vi "SLL DE Get DO Safe Values form INI File.vi"(8 "error in (no error)":errorcluster) -> (0 "error out":errorcluster, 1 "DO Safe Values":bool[](array[boolean]), 2 "DO Channel Names (String)":string[](array[string]), 3 "DO Channels (Enum)":T1[](array[typedef]))   [LabVIEW 2013]
doc: "Copyright © 2005, Soliton Technologies.\nAll rights reserved."
uses:
  Controls/SLL DE List of Digital Outputs.ctl
  Controls/SLL DE DAQ Parameters LV2Global Options.ctl
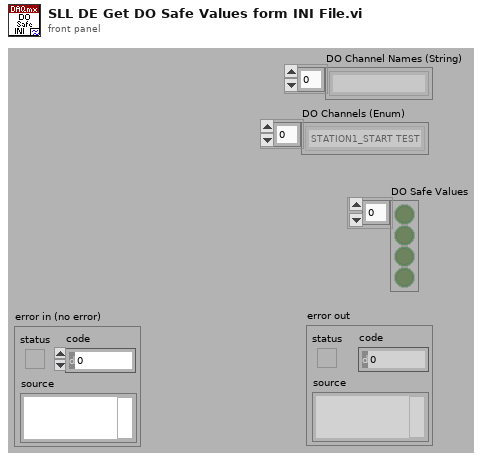
[diagram p1: front panel]
types:
  T1 = typedef "SLL DE List of Digital Outputs.ctl" = enum16{"STATION1_START TEST", "STATION1_STOP TEST", "STATION1_LIGHT1", "STATION1_LIGHT2", "STATION1_LIGHT3", "STATION1_SELECT_TEST", "STATION2_START TEST", "STATION2_STOP TEST", "STATION2_LIGHT1", "STATION2_LIGHT2", "STATION2_LIGHT3", "STATION2_SELECT_TEST", "STATION3_START TEST", "STATION3_STOP TEST", "STATION3_LIGHT1", "STATION3_LIGHT2", "STATION3_LIGHT3", "STATION3_SELECT_TEST", "STATION4_START TEST", "STATION4_STOP TEST", "STATION4_LIGHT1", "STATION4_LIGHT2", "STATION4_LIGHT3", "STATION4_SELECT_TEST"}
  T2 = typedef "SLL DE DAQ Parameters LV2Global Options.ctl" = enum16{"Read", "Write"}
  T3 = typedef "SLL DE DAQ Engine Parameters.ctl" = cluster{"Enable Engines":cluster{"AI Enable":bool, "AO Enable":bool, "DI Enable":bool, "DO Enable":bool}, "DAQ Control Type":cluster{"Analog Input":enum16{"Finite", "Continuous", "Driver"}, "Analog Output":enum16{"Finite", "Continuous", "Driver"}, "Digital Input":enum16{"Finite", "Continuous", "Driver"}, "Digital Output":enum16{"Finite", "Continuous", "Driver"}}, "DAQ Parameters":cluster{"AI Sampling Rate (Samples/Sec)":dbl, "MvgAVG Window Size (# of Points)":i32, "Enable Filter":bool, "Enable MvgAVG":bool, "Circular Buffer Size (Sec)":dbl, "AO Sampling Rate (Samples/Sec)":dbl, "Graph Update Rate (Samples/Sec)":dbl, "File Logging Rate (Samples/Sec)":i32}, "AO Safe Values":cluster{"Analog Outputs Name":T4, "Analog Outputs Safe Value":dbl}[], "DO Safe Values":cluster{"Digital Outputs Name":T1, "Digital Outputs Safe Value":bool}[], "DO Interconnected Lines":cluster{"First DO Line":string, "Second DO Line":string}[], "AI Channels Unit":cluster{"Channel Name":T5, "Channel Type":T6}[], "Units Information":cluster{"Channel Type":T6, "Unit Text":string, "Maximum":dbl, "Minmum":dbl, "Increments":dbl}[]}
  T4 = typedef "SLL DE List of Analog Outputs.ctl" = enum16{"None"}
  T5 = typedef "SLL DE List of Analog Inputs.ctl" = enum16{"None"}
  T6 = typedef "SLL DE List of AI Channel Type.ctl" = enum16{"Pressure", "Flow", "Temperature", "Time Scale", "Voltage", "Current", "Frequency", "Sound", "Speed", "Torque", "Distance", "Channel Type 1", "Channel Type 2", "Channel Type 3"}
  T7 = cluster{"Digital Outputs Name":T1, "Digital Outputs Safe Value":bool}[]
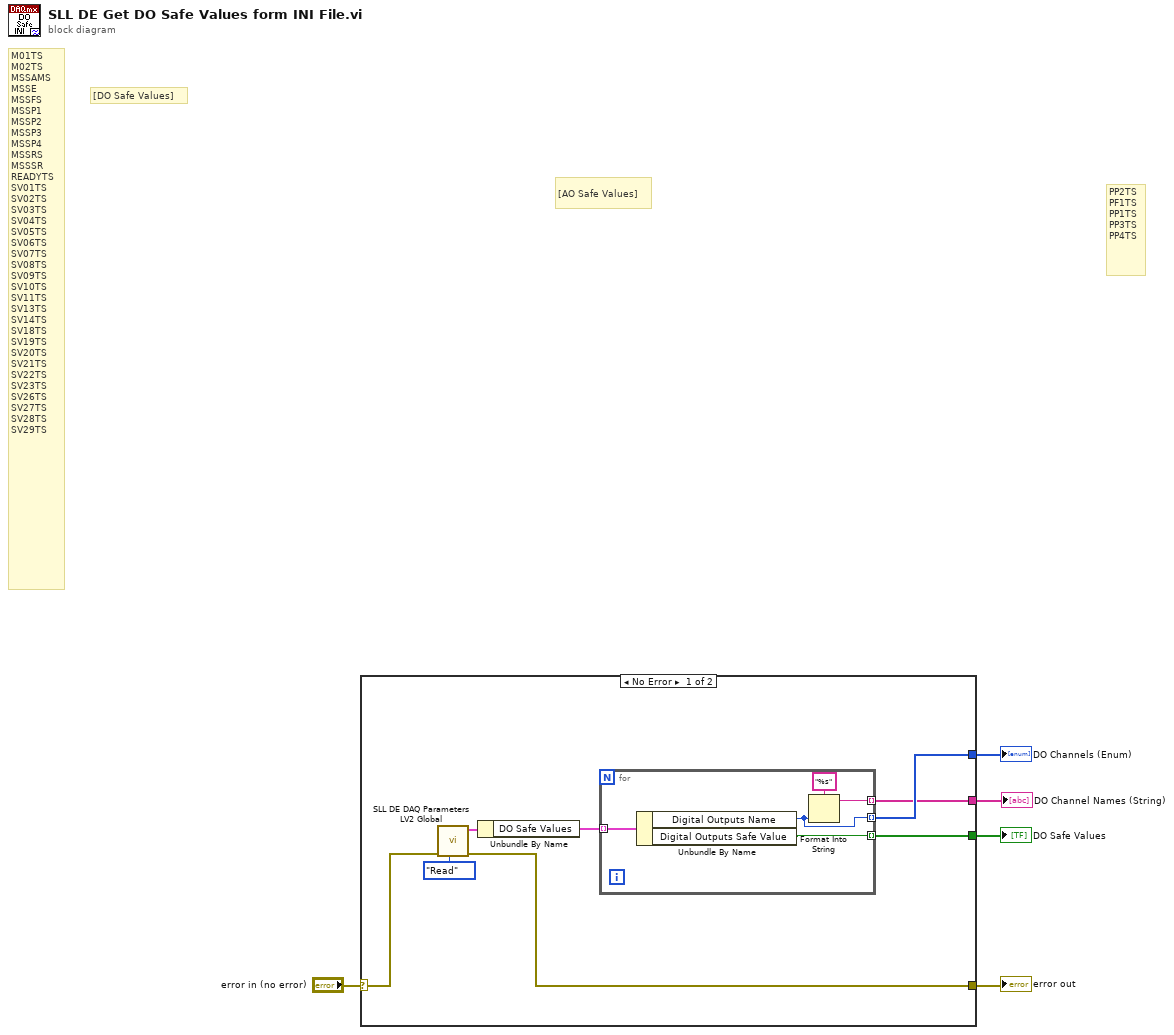
[diagram p0: block diagram]
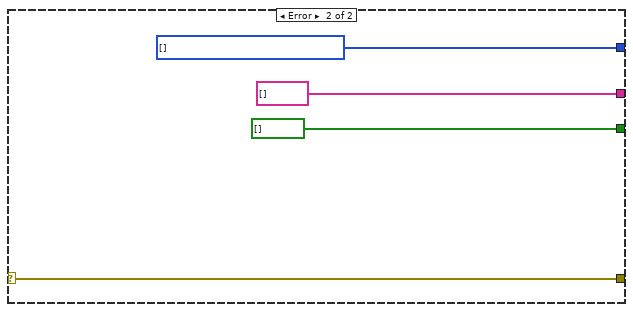
[diagram p2: hidden frame]
diagram:
  # "[DO Safe Values]"
  # "PP2TS\nPF1TS\nPP1TS\nPP3TS\nPP4TS"
  # "[AO Safe Values]"
  # "M01TS\nM02TS\nMSSAMS\nMSSE\nMSSFS\nMSSP1\nMSSP2\nMSSP3\nMSSP4\nMSSRS\nMSSSR\nREADYTS\nSV01TS\nSV02TS\nSV03TS\nSV04TS\nSV05TS\nSV06TS\nSV07TS\nSV08TS\nSV09TS\nSV10TS\nSV11TS\nSV13TS\nSV14TS\nSV18TS\nSV19TS\nSV20TS\nSV21TS\nSV22TS\nSV23TS\nSV26TS\nSV27TS\nSV28TS\nSV29TS"
  n1 = case shown="No Error" "error in (no error)" {
    selector: "error in (no error)" -> [w13 w22]
    tunnel: [w12 w22] -> w4
    tunnel: [w11 bool[] [] ("Key Values")] -> w3
    tunnel: [w10 w20] -> w2
    tunnel: [w9 string[] []] -> w1
    frame No Error {
      n2 = call "SLL DE DAQ Parameters LV2 Global.vi"("Option"=SLL_DE_DAQ_Parameters_LV2Global_Options."Read", "Error in (no error)"=w13) -> ("Error out"=w12:errorcluster, "Global Info"=w7:T3)  [unwired: 8 in]
      n3 = Unbundle By Name(w7) -> ("DO Safe Values"=w8:T7)
      n4 = for {
        tunnel: w8 -> [w18] mode=indexing
        tunnel: [w16] -> w11 mode=indexing
        tunnel: [w15] -> w10 mode=indexing
        tunnel: [w14] -> w9 mode=indexing
        n5 = Unbundle By Name(w18) -> ("Digital Outputs Name"=w15:T1, "Digital Outputs Safe Value"=w16:bool)
        n6 = Format Into String(format string="%s", w15) -> (resulting string=w14:string)  [unwired: 2 in, 1 out]
      }
    }
    frame Error {
      w20 = T1[] [] items=["STATION1_START TEST", "STATION1_STOP TEST", "STATION1_LIGHT1", "STATION1_LIGHT2", "STATION1_LIGHT3", "STATION1_SELECT_TEST", "STATION2_START TEST", "STATION2_STOP TEST", "STATION2_LIGHT1", "STATION2_LIGHT2", "STATION2_LIGHT3", "STATION2_SELECT_TEST", "STATION3_START TEST", "STATION3_STOP TEST", "STATION3_LIGHT1", "STATION3_LIGHT2", "STATION3_LIGHT3", "STATION3_SELECT_TEST", "STATION4_START TEST", "STATION4_STOP TEST", "STATION4_LIGHT1", "STATION4_LIGHT2", "STATION4_LIGHT3", "STATION4_SELECT_TEST"]
    }
  }
  "error out" <- w4
  "DO Safe Values" <- w3
  "DO Channels (Enum)" <- w2
  "DO Channel Names (String)" <- w1
